vi "Get Path Transformations.vi"(8 "error in (no error)":errorcluster, 11 "NI_AB_API_Build in":refnum<class "NI_AB_API_Build.lvclass">) -> (0 "error out":errorcluster, 1 "New Paths":path[](array[path]), 2 "Original Paths":path[](array[path]), 3 "NI_AB_API_Build out":refnum<class "NI_AB_API_Build.lvclass">)   [LabVIEW 2020, in "NI_AB_API_Build.lvclass"]
uses:
  <vilib>/AppBuilder/AB_API/Build/NI_AB_API_Build.lvclass
  <vilib>/AppBuilder/AB_API/Build/NI_AB_API_Build.lvclass/NI_AB_API_Build.ctl
  <vilib>/AppBuilder/AB_Classes/Build/AB_Build.lvclass
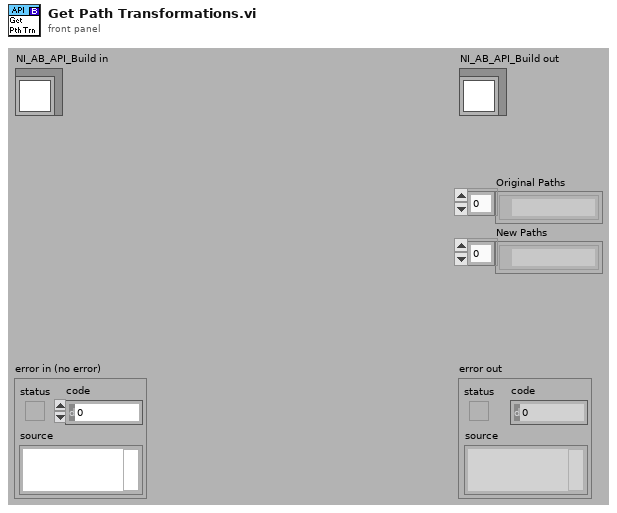
[diagram p1: front panel]
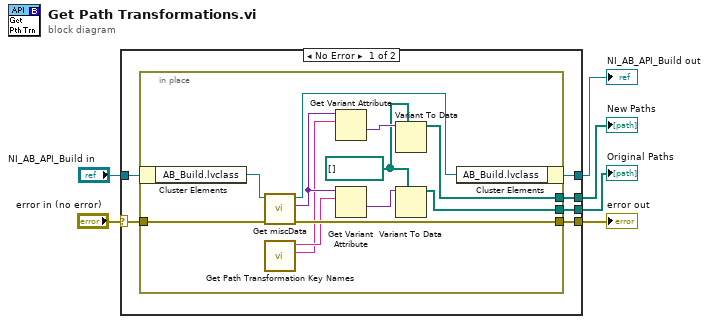
[diagram p0: block diagram]
diagram:
  n1 = case shown="No Error" "error in (no error)" {
    selector: "error in (no error)" -> [w12 w26]
    tunnel: [w11 w26] -> w5
    tunnel: [w7 w25] -> w3
    tunnel: "NI_AB_API_Build in" -> [w8 w25]
    tunnel: [w10 _] -> w2
    tunnel: [w9 _] -> w1
    frame No Error {
      n2 = in-place {
        in-place-border: w12 -> [w24]
        in-place-border: [w23] -> w11
        in-place-border: [w22] -> w10
        in-place-border: [w21] -> w9
        w15 = path[] [] ("Broken VI List")
        n3 = in-place-cluster #1(w8) -> ("AB_Build.lvclass"=w14:refnum<class "AB_Build.lvclass">)
        n4 = call-dynamic "Get miscData.vi"("error in (no error)"=w24, "AB_Build in"=w14) -> ("error out"=w23:errorcluster, "eng_miscData"=w19:variant, "AB_Build out"=w13:refnum<class "AB_Build.lvclass">)  [unwired: 7 in]
        n5 = call <vilib>:"Get Path Transformation Key Names.vi"() -> ("New Paths Key"=w16:string, "Original Paths Key"=w17:string)  [unwired: 9 in, 1 out]
        n6 = Get Variant Attribute(Variant=w19, name=w16) -> (value=w18:variant)  [unwired: 2 in, 3 out]
        n7 = Get Variant Attribute(Variant=w19, name=w17) -> (value=w20:variant)  [unwired: 2 in, 3 out]
        n8 = Variant To Data(type=w15, Variant=w18) -> (data=w21:path[])  [unwired: 1 in, 1 out]
        n9 = Variant To Data(type=w15, Variant=w20) -> (data=w22:path[])  [unwired: 1 in, 1 out]
        n10 = in-place-cluster #1("AB_Build.lvclass"=w13) -> (w7:refnum<class "NI_AB_API_Build.lvclass">)
      }
    }
    frame Error {
    }
  }
  "error out" <- w5
  "NI_AB_API_Build out" <- w3
  "Original Paths" <- w2
  "New Paths" <- w1
